vi "GameToIAStateOffensive.vi"(8 "error in (no error)":errorcluster, 11 "Game in":refnum<class "Game.lvclass">) -> (0 "error out":errorcluster, 1 "RobotRef":refnum<class "Robot.lvclass">[](array[class]), 2 "IA State out":T1={"our_robots"=[], "enemy_robots"=[], "balls"=[], "geometry"={"line_width"=0, "field_length"=0, "field_width"=0, "boundary_width"=0, "referee_width"=0, "goal_width"=0, "goal_depth"=0, "goal_wall_width"=0, "center_circle_radius"=0, "defense_radius"=0, "defense_stretch"=0, "free_kick_from_defense_dist"=0, "penalty_spot_from_field_line_dist"=0, "penalty_line_from_spot_dist"=0}, "IA Judge"={"stage"="", "command"="", "our_goalie_id"=0.0, "enemy_goalie_id"=0.0, "command enum"=enum."Halt", "Time"=enum."Azul"}, "Received Timestamp"=timestamp(0 s since 1904-01-01), "Events"={"Touch"=FALSE, "Ball out"=FALSE, "id touch"=0.0, "Ball out of \nVision"=FALSE, "Ball inside \nGoalie area"=FALSE, "Robot not responding"=FALSE, "Robots responding status"=[1.0, 1.0, 1.0, 1.0, 1.0, 1.0], "Enemy Ball \nPossession"=FALSE, "Pass State"=FALSE, "id end of pass"=0.0, "Kick"=FALSE, "Id ini Possession"=0.0, "Ball Possesion"=FALSE, "Id Possesion"=0.0, "Direct Kick"=FALSE, "2nd Strk Ativo"=FALSE}}, 3 "Game out":refnum<class "Game.lvclass">)   [LabVIEW 2018, in "Game.lvclass"]
uses:
  Game.lvclass
  Vision_class/Old vision/SSL Detection Frame Simple Estimator Cameras VelCmd Folder/Core/AI Input.ctl
  Communication_class/Paths/Convert AI Robot to Robot Command Folder/Core/AI Robot.ctl
  Communication_class/Paths/Convert AI Robot to Robot Command Folder/Intel/Functions Enum.ctl
  Communication_class/Paths/Convert AI Robot to Robot Command Folder/Intel/AttackerStates.ctl
  Communication_class/Paths/Convert AI Robot to Robot Command Folder/Path Planning/RRT/PathDests.ctl
  Communication_class/Paths/Convert AI Robot to Robot Command Folder/Path Planning/RRT/PathDest.ctl
  Communication_class/Paths/MessageAI_State Folder/Core/AI Ball.ctl
  Communication_class/Paths/MessageAI_State Folder/Core/Field Size.ctl
  Vision_class/Old vision/SSL Detection Frame Simple Estimator Cameras VelCmd Folder/Core/AI Judge.ctl
  Communication_class/Paths/MessageAI_State Folder/Intel/Command Enum.ctl
  Vision_class/Old vision/SSL Detection Frame Simple Estimator Cameras VelCmd Folder/Util/Events/Events.ctl
  Robot_class/Robot.lvclass
  Team_class/OffensivePlay.ctl
  Game.lvclass/Game.ctl
  Team_class/Team.lvclass/Team.ctl
  Object_class/Object.lvclass/Object.ctl
  Ball_class/Ball.lvclass/Ball.ctl
  Events_class/Events.lvclass/Events.ctl
  Referee_class/Referee.lvclass/Referee.ctl
  Robot_class/Robot.lvclass/Robot.ctl
  Robot_class/Read id.vi
  Object_class/Read x.vi
  Object_class/Read y.vi
  Robot_class/Read orientation.vi
  Robot_class/Read est_v_tang.vi
  Robot_class/Read est_v_norm.vi
  Object_class/Read pos_est_x.vi
  Object_class/Read pos_est_y.vi
  Robot_class/Read dribble.vi
  Robot_class/Read path.vi
  Robot_class/Read path_smooth.vi
  Robot_class/Read dest_x.vi
  Robot_class/Read dest_y.vi
  Robot_class/Read dest_orientation.vi
  Read OffensiveTeam.vi
  Read EnemyRef.vi
  Read BallRef.vi
  Read EventsRef.vi
  Read FieldRef.vi
  Read Referee.vi
  Read TimeRef.vi
  Referee_class/Read command_from_referee.vi
  Referee_class/Read command_interpreted.vi
  Events_class/Read ball_inside_enemy_goalie_area.vi
  Events_class/Read ball_inside_our_goalie_area.vi
  Events_class/Read ball_out.vi
  Events_class/Read ball_out_of_vision.vi
  Events_class/Read enemy_ball_possesion.vi
  Events_class/Read id_enemy_ball_possesion.vi
  Events_class/Read id_our_balll_possesion.vi
  Events_class/Read id_touch.vi
  Events_class/Read kick.vi
  Events_class/Read our_balll_possesion.vi
  Events_class/Read touch.vi
  Ball_class/Read v_x.vi
  Ball_class/Read v_y.vi
  Team_class/Read RobotRef.vi
  Team_class/Read OffensivePlay.vi
  Ball_class/Ball.lvclass
  Enemy_class/Enemy.lvclass
  Ally_class/Ally.lvclass
  Events_class/Events.lvclass
  Field_class/Field.lvclass
  Referee_class/Referee.lvclass
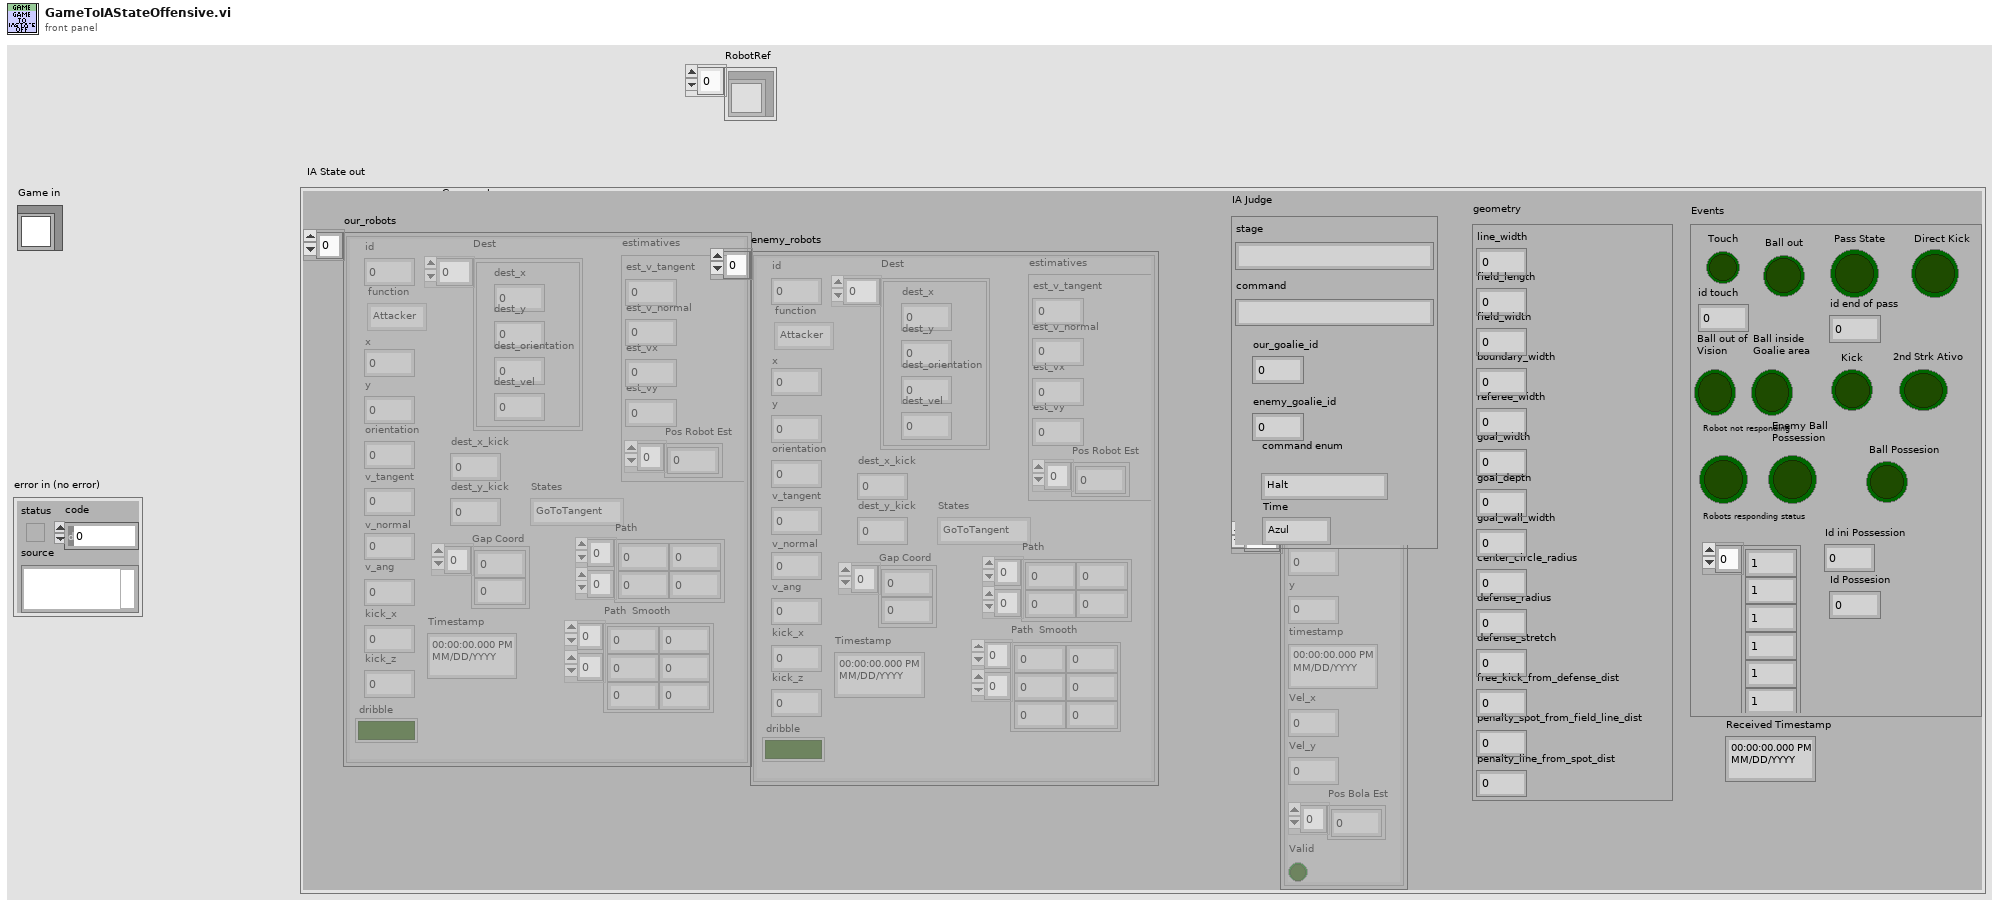
[diagram p1: front panel]
types:
  T1 = typedef "AI Input.ctl" = cluster{"our_robots":T2[], "enemy_robots":T2[], "balls":T7[], "geometry":T8, "IA Judge":T9, "Received Timestamp":timestamp, "Events":T11}
  T2 = typedef "AI Robot.ctl" = cluster{"id":u32, "function":T3, "x":dbl, "y":dbl, "orientation":dbl, "v_tangent":dbl, "v_normal":dbl, "v_ang":dbl, "kick_x":dbl, "kick_z":dbl, "dribble":bool, "Timestamp":timestamp, "estimatives":cluster{"est_v_tangent":dbl, "est_v_normal":dbl, "est_vx":dbl, "est_vy":dbl, "Pos Robot Est":dbl[]}, "dest_x_kick":dbl, "dest_y_kick":dbl, "Gap Coord":dbl[], "States":T4, "Path ":dbl[][], "Path  Smooth":dbl[][], "Dest":T5}
  T3 = typedef "Functions Enum.ctl" = enum16{"2nd Striker", "Attacker", "Goalie", "Defender", "Striker", "Goto 0", "Dummy", "Kicker", "ZigZag 0", "ZigZag 1", "ZigZag 2", "ZigZag 3", "ZigZag 4", "ZigZag 5", "ZigZag 6", "ZigZag 7", "ZigZag 8", ""}
  T4 = typedef "AttackerStates.ctl" = enum16{"Pass", "GoToTangent", "BallGetting", "GoToKick", ""}
  T5 = typedef "PathDests.ctl" = T6[]
  T6 = typedef "PathDest.ctl" = cluster{"dest_x":dbl, "dest_y":dbl, "dest_orientation":dbl, "dest_vel":dbl}
  T7 = typedef "AI Ball.ctl" = cluster{"x":dbl, "y":dbl, "timestamp":timestamp, "Vel_x":dbl, "Vel_y":dbl, "Pos Bola Est":dbl[], "Valid":bool}
  T8 = typedef "Field Size.ctl" = cluster{"line_width":u32, "field_length":u32, "field_width":u32, "boundary_width":u32, "referee_width":u32, "goal_width":u32, "goal_depth":u32, "goal_wall_width":u32, "center_circle_radius":u32, "defense_radius":u32, "defense_stretch":u32, "free_kick_from_defense_dist":u32, "penalty_spot_from_field_line_dist":u32, "penalty_line_from_spot_dist":u32}
  T9 = typedef "AI Judge.ctl" = cluster{"stage":string, "command":string, "our_goalie_id":dbl, "enemy_goalie_id":dbl, "command enum":T10, "Time":enum16{"Azul", "Amarelo"}}
  T10 = typedef "Command Enum.ctl" = enum16{"Halt", "Stop", "Force Start", "PKA Normal Start", "Prepare Kickoff Ally", "PKE Normal Start", "Prepare Kickoff Enemy", "Prepare Penalty Ally", "PPA Normal Start", "Prepare Penalty Enemy", "PPE Normal Start", "Direct Free Enemy", "Direct Free Ally", "Indirect Free Enemy", "Indirect Free Ally", "Timeout Enemy", "Timeout Ally", "Goal Enemy", "Goal Ally", "Ball Placement Enemy", "Ball Placement Ally", "Normal Half Time", "Extra Time Break", "Extra Half Time", "None", "Post Game"}
  T11 = typedef "Events.ctl" = cluster{"Touch":bool, "Ball out":bool, "id touch":dbl, "Ball out of \nVision":bool, "Ball inside \nGoalie area":bool, "Robot not responding":bool, "Robots responding status":dbl[], "Enemy Ball \nPossession":bool, "Pass State":bool, "id end of pass":dbl, "Kick":bool, "Id ini Possession":dbl, "Ball Possesion":bool, "Id Possesion":dbl, "Direct Kick":bool, "2nd Strk Ativo":bool}
  T12 = typedef "OffensivePlay.ctl" = enum16{"PreparePass", "PassToStriker", "BallOutOfField", "PassTo2ndStriker", "StopOffensive", "Prepare Penalty Enemy", "EnemyPossessionAtEnemyField", "EnemyPossesionAtOurField", "TestPlay", "PreparePenaltyAlly", "KickPenaltyAlly", "PrepareKickoffAlly", "PrepareKickoffEnemy", "IndirectEnemy", "DirectEnemy", "NormalGame", "DirectKick", "Pass", "Halt", "Timeout", "PassPlay", "PenaltyEnemy"}
  T13 = typedef "command_interpreted.ctl" = enum16{"Goal Ally", "Goal Enemy", "Ball Placement Enemy", "Ball Placement Ally", "Normal Half Time", "Extra Time  Break", "Extra Half Time", "None", "Post Game", "PKA Normal Start", "Prepare Kickoff Ally", "PKE Normal Start", "Prepare Kickoff Enemy", "Force Start", "Halt", "Timeout", "Prepare Penalty Ally", "Prepare Penalty Enemy", "PPA NormalStart", "PPE Normal Start", "Indirect Free Ally", "Direct Free Enemy", "Direct Free Ally", "Indirect Free Enemy", "Stop"}
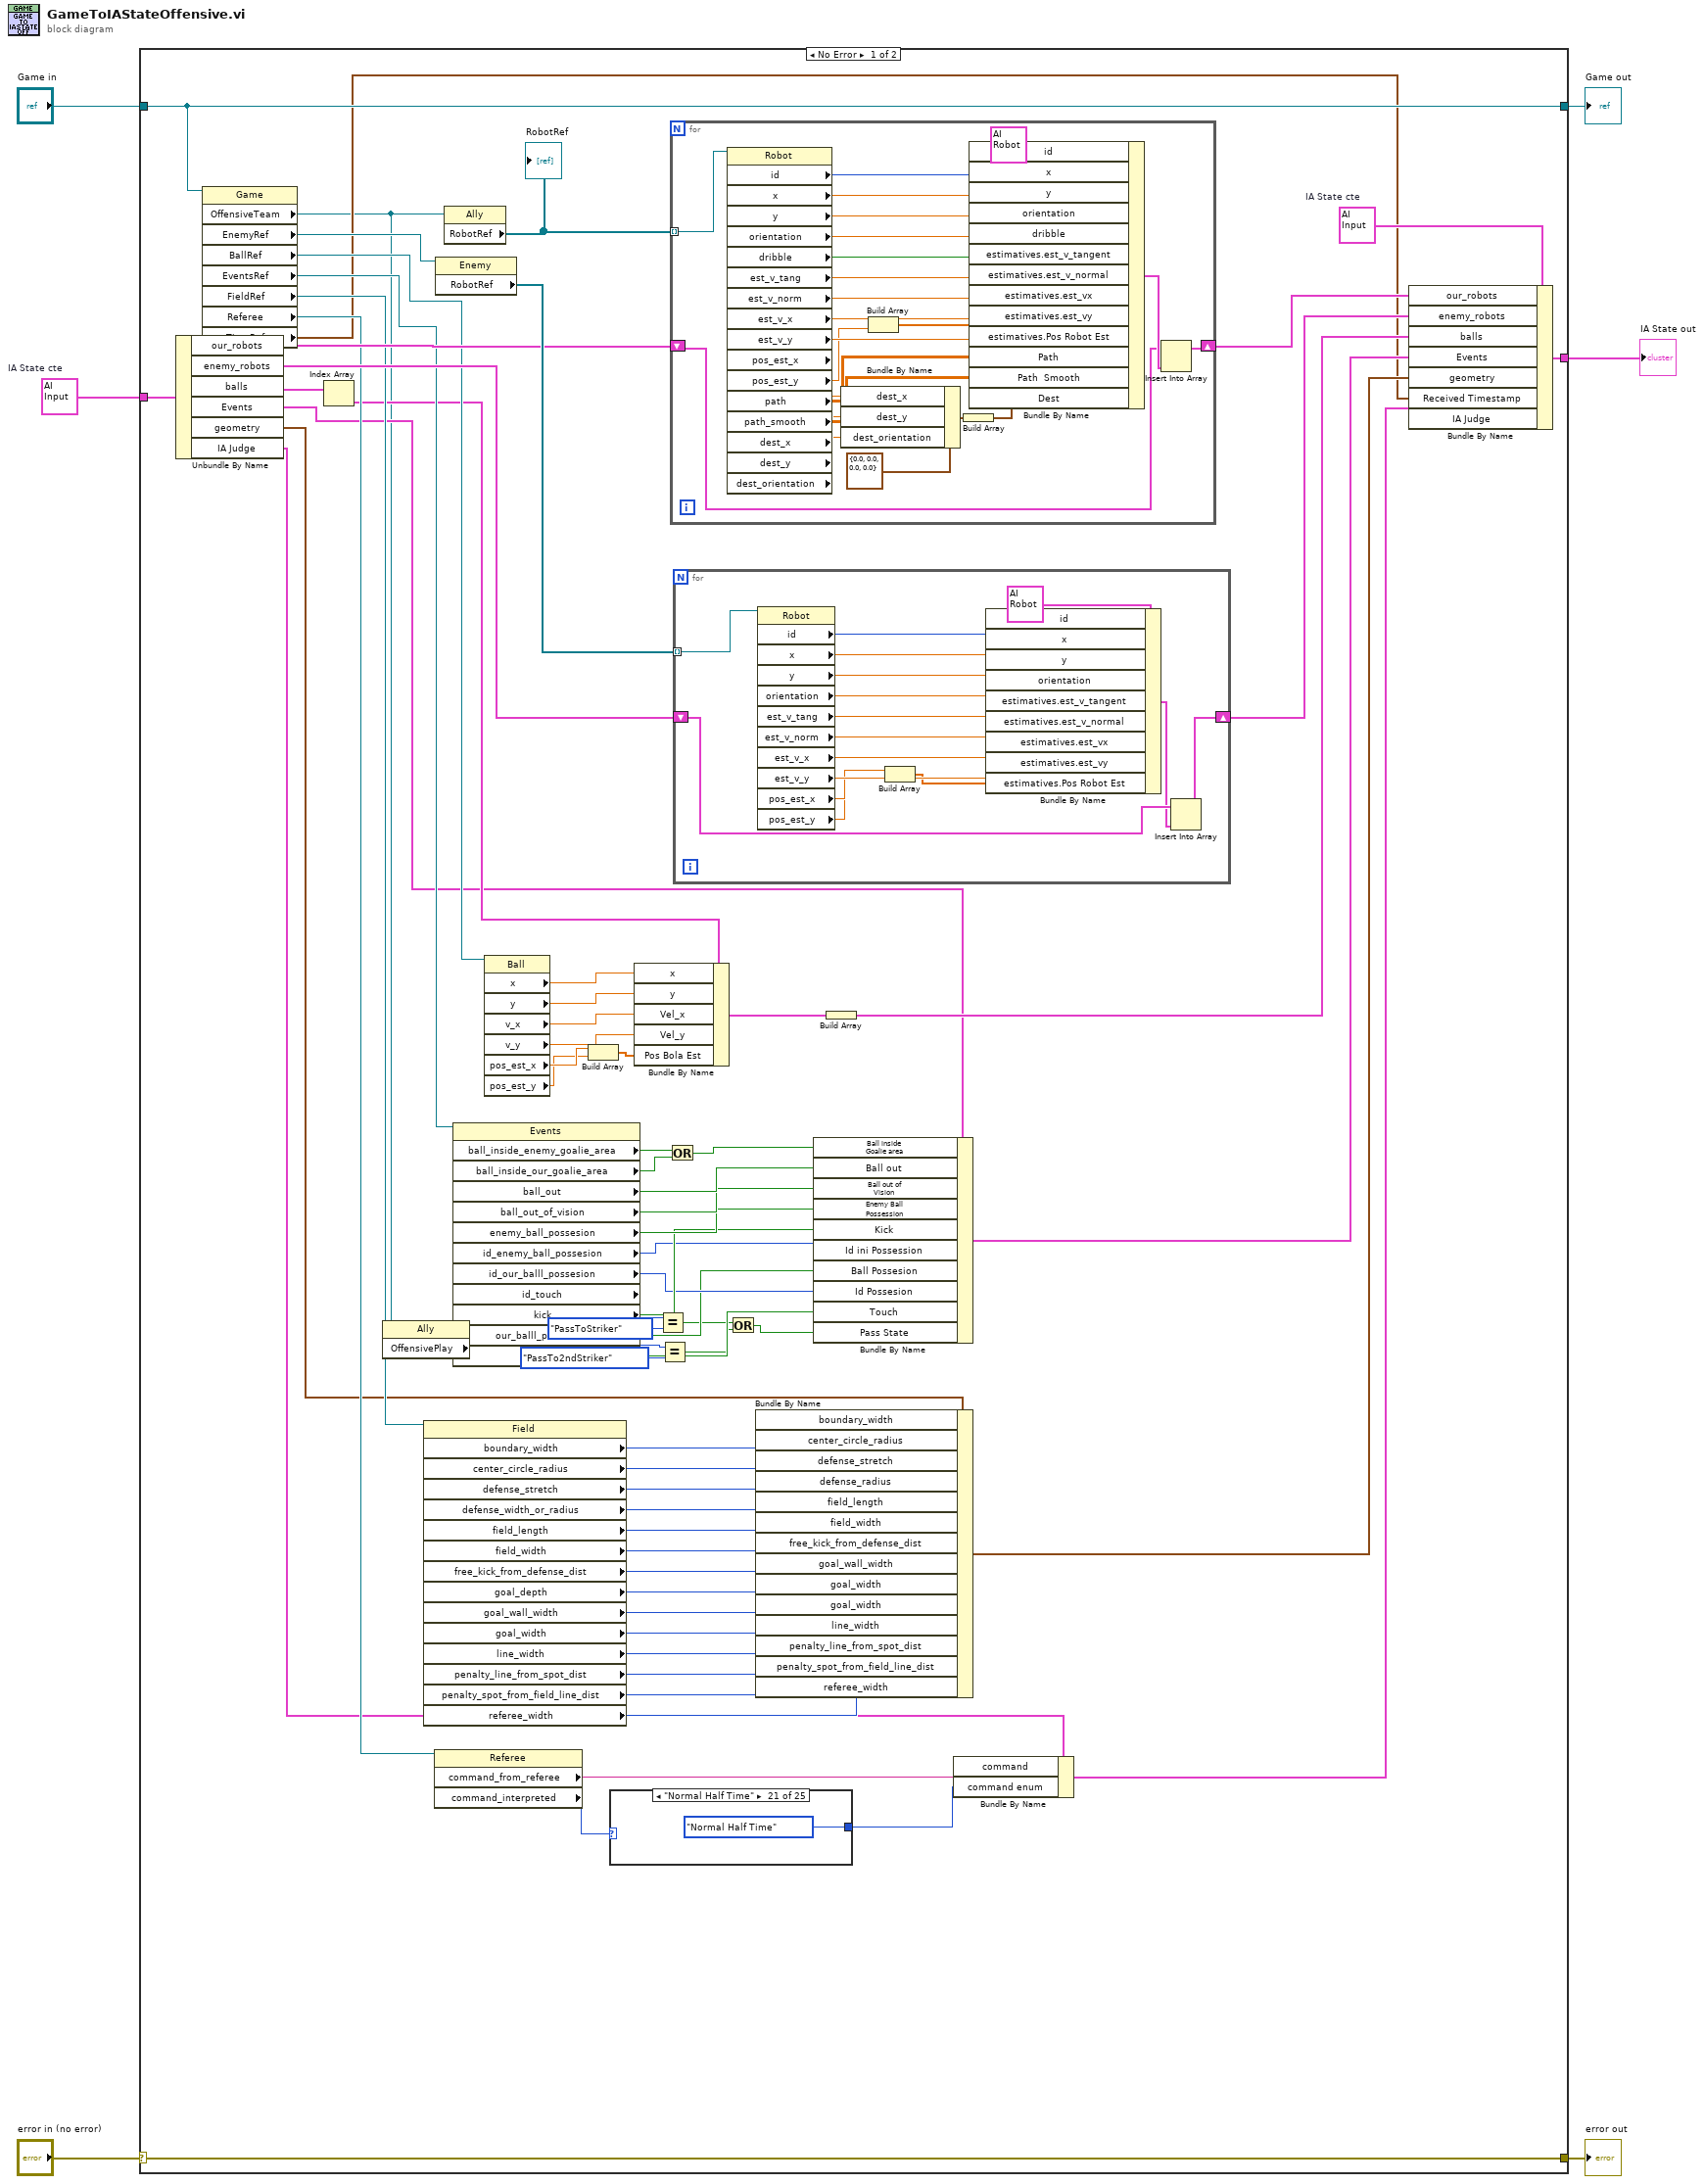
[diagram p0: block diagram]
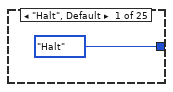
[diagram p2: hidden frame]
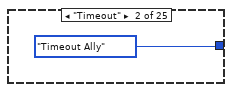
[diagram p3: hidden frame]
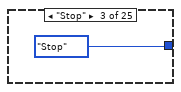
[diagram p4: hidden frame]
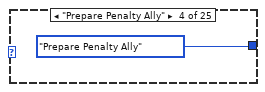
[diagram p5: hidden frame]
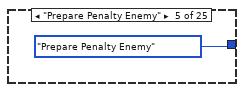
[diagram p6: hidden frame]
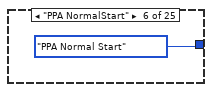
[diagram p7: hidden frame]
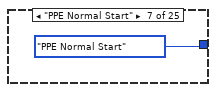
[diagram p8: hidden frame]
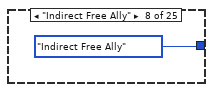
[diagram p9: hidden frame]
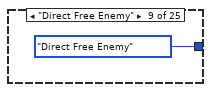
[diagram p10: hidden frame]
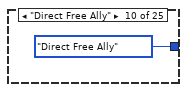
[diagram p11: hidden frame]
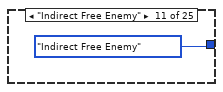
[diagram p12: hidden frame]
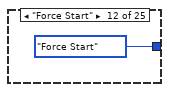
[diagram p13: hidden frame]
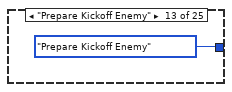
[diagram p14: hidden frame]
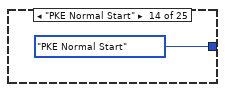
[diagram p15: hidden frame]
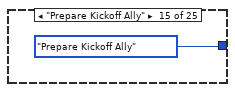
[diagram p16: hidden frame]
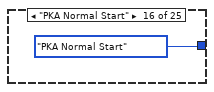
[diagram p17: hidden frame]
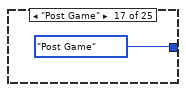
[diagram p18: hidden frame]
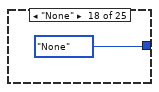
[diagram p19: hidden frame]
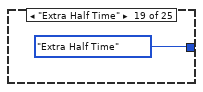
[diagram p20: hidden frame]
diagram:
  w2 = T1 {"our_robots"=[], "enemy_robots"=[], "balls"=[], "geometry"={"line_width"=0, "field_length"=0, "field_width"=0, "boundary_width"=0, "referee_width"=0, "goal_width"=0, "goal_depth"=0, "goal_wall_width"=0, "center_circle_radius"=0, "defense_radius"=0, "defense_stretch"=0, "free_kick_from_defense_dist"=0, "penalty_spot_from_field_line_dist"=0, "penalty_line_from_spot_dist"=0}, "IA Judge"={"stage"="", "command"="", "our_goalie_id"=0.0, "enemy_goalie_id"=0.0, "command enum"=enum."Halt", "Time"=enum."Azul"}, "Received Timestamp"=timestamp(0 s since 1904-01-01), "Events"={"Touch"=FALSE, "Ball out"=FALSE, "id touch"=0.0, "Ball out of \nVision"=FALSE, "Ball inside \nGoalie area"=FALSE, "Robot not responding"=FALSE, "Robots responding status"=[], "Enemy Ball \nPossession"=FALSE, "Pass State"=FALSE, "id end of pass"=0.0, "Kick"=FALSE, "Id ini Possession"=0.0, "Ball Possesion"=FALSE, "Id Possesion"=0.0, "Direct Kick"=FALSE, "2nd Strk Ativo"=FALSE}}  # IA State cte
  n1 = case shown="No Error" "error in (no error)" {
    selector: "error in (no error)" -> [w75 w144]
    tunnel: [w75 w144] -> w5
    tunnel: [w74 w143] -> w3
    tunnel: "Game in" -> [w74 w143]
    tunnel: w2 -> [w70 w142]
    tunnel: [w14 w142] -> w1
    frame No Error {
      w66 = T1 {"our_robots"=[], "enemy_robots"=[], "balls"=[], "geometry"={"line_width"=0, "field_length"=0, "field_width"=0, "boundary_width"=0, "referee_width"=0, "goal_width"=0, "goal_depth"=0, "goal_wall_width"=0, "center_circle_radius"=0, "defense_radius"=0, "defense_stretch"=0, "free_kick_from_defense_dist"=0, "penalty_spot_from_field_line_dist"=0, "penalty_line_from_spot_dist"=0}, "IA Judge"={"stage"="", "command"="", "our_goalie_id"=0.0, "enemy_goalie_id"=0.0, "command enum"=enum."Halt", "Time"=enum."Azul"}, "Received Timestamp"=timestamp(0 s since 1904-01-01), "Events"={"Touch"=FALSE, "Ball out"=FALSE, "id touch"=0.0, "Ball out of \nVision"=FALSE, "Ball inside \nGoalie area"=FALSE, "Robot not responding"=FALSE, "Robots responding status"=[], "Enemy Ball \nPossession"=FALSE, "Pass State"=FALSE, "id end of pass"=0.0, "Kick"=FALSE, "Id ini Possession"=0.0, "Ball Possesion"=FALSE, "Id Possesion"=0.0, "Direct Kick"=FALSE, "2nd Strk Ativo"=FALSE}}  # IA State cte
      n2 = Unbundle By Name(w70) -> ("our_robots"=w69:T2[], "enemy_robots"=w68:T2[], "balls"=w23:T7[], "Events"=w21:T11, "geometry"=w20:T8, "IA Judge"=w18:T9)
      n3 = property class="Game"(reference=w74) -> ("OffensiveTeam"=w13:refnum<class "Ally.lvclass">, "EnemyRef"=w72:refnum<class "Enemy.lvclass">, "BallRef"=w67:refnum<class "Ball.lvclass">, "EventsRef"=w54:refnum<class "Events.lvclass">, "FieldRef"=w41:refnum<class "Field.lvclass">, "Referee"=w25:refnum<class "Referee.lvclass">, "TimeRef"=w19:timestamp)  [unwired: 1 in, 2 out]
      n4 = Index Array(array=w23) -> (element=w22:T7)  [unwired: 1 in]
      n5 = property class="Ally"(reference=w13) -> ("OffensivePlay"=w9:T12)  [unwired: 1 in, 2 out]
      n6 = property class="Field"(reference=w41) -> ("boundary_width"=w40:i32, "center_circle_radius"=w39:i32, "defense_stretch"=w38:i32, "defense_width_or_radius"=w37:i32, "field_length"=w36:i32, "field_width"=w35:i32, "free_kick_from_defense_dist"=w34:i32, "goal_depth"=w33:i32, "goal_wall_width"=w32:i32, "goal_width"=w31:i32, "line_width"=w30:i32, "penalty_line_from_spot_dist"=w29:i32, "penalty_spot_from_field_line_dist"=w28:i32, "referee_width"=w27:i32)  [unwired: 1 in, 2 out]
      n7 = property class="Referee"(reference=w25) -> ("command_from_referee"=w24:string, "command_interpreted"=w17:T13)  [unwired: 1 in, 2 out]
      n8 = property class="Enemy"(reference=w72) -> ("RobotRef"=w71:refnum<class "Robot.lvclass">[])  [unwired: 1 in, 2 out]
      n9 = property class="Ally"(reference=w13) -> ("RobotRef"=w73:refnum<class "Robot.lvclass">[])  [unwired: 1 in, 2 out]
      "RobotRef" <- w73
      n10 = property class="Events" props=["ball_inside_enemy_goalie_area", "ball_inside_our_goalie_area", "ball_out", "ball_out_of_vision", "enemy_ball_possesion", "id_enemy_ball_possesion", "id_our_balll_possesion", "id_touch", "kick", "our_balll_possesion", "touch"](reference=w54) -> ("ball_inside_enemy_goalie_area"=w52:bool, "ball_inside_our_goalie_area"=w53:bool, "ball_out"=w50:bool, "ball_out_of_vision"=w49:bool, "enemy_ball_possesion"=w48:bool, "id_enemy_ball_possesion"=w46:i32, "id_our_balll_possesion"=w45:i32, "kick"=w47:bool, "our_balll_possesion"=w44:bool, "touch"=w43:bool)  [unwired: 1 in, 3 out]
      n11 = property class="Ball"(reference=w67) -> ("x"=w63:dbl, "y"=w62:dbl, "v_x"=w61:dbl, "v_y"=w60:dbl, "pos_est_x"=w59:dbl, "pos_est_y"=w58:dbl)  [unwired: 1 in, 2 out]
      n12 = Build Array(w59, w58) -> (w57:dbl[])
      n13 = case shown="\"Normal Half Time\"" w17 {
        tunnel: [Command_Enum."Halt" ("command enum") Command_Enum."Timeout Ally" ("command enum") Command_Enum."Stop" ("command enum") Command_Enum."Prepare Penalty Ally" ("command enum") Command_Enum."Prepare Penalty Enemy" ("command enum") Command_Enum."PPA Normal Start" ("command enum") Command_Enum."PPE Normal Start" ("command enum") Command_Enum."Indirect Free Ally" ("command enum") Command_Enum."Direct Free Enemy" ("command enum") Command_Enum."Direct Free Ally" ("command enum") Command_Enum."Indirect Free Enemy" ("command enum") Command_Enum."Force Start" ("command enum") Command_Enum."Prepare Kickoff Enemy" ("command enum") Command_Enum."PKE Normal Start" ("command enum") Command_Enum."Prepare Kickoff Ally" ("command enum") Command_Enum."PKA Normal Start" ("command enum") Command_Enum."Post Game" ("command enum") Command_Enum."None" ("command enum") Command_Enum."Extra Half Time" ("command enum") Command_Enum."Extra Time Break" ("command enum") Command_Enum."Normal Half Time" ("command enum") Command_Enum."Ball Placement Ally" ("command enum") Command_Enum."Ball Placement Enemy" ("command enum") Command_Enum."Goal Enemy" ("command enum") Command_Enum."Goal Ally" ("command enum")] -> w16
        frame "Halt", Default {
        }
        frame "Timeout" {
        }
        frame "Stop" {
        }
        frame "Prepare Penalty Ally" {
        }
        frame "Prepare Penalty Enemy" {
        }
        frame "PPA NormalStart" {
        }
        frame "PPE Normal Start" {
        }
        frame "Indirect Free Ally" {
        }
        frame "Direct Free Enemy" {
        }
        frame "Direct Free Ally" {
        }
        frame "Indirect Free Enemy" {
        }
        frame "Force Start" {
        }
        frame "Prepare Kickoff Enemy" {
        }
        frame "PKE Normal Start" {
        }
        frame "Prepare Kickoff Ally" {
        }
        frame "PKA Normal Start" {
        }
        frame "Post Game" {
        }
        frame "None" {
        }
        frame "Extra Half Time" {
        }
        frame "Extra Time  Break" {
        }
        frame "Normal Half Time" {
        }
        frame "Ball Placement Ally" {
        }
        frame "Ball Placement Enemy" {
        }
        frame "Goal Enemy" {
        }
        frame "Goal Ally" {
        }
      }
      n14 = Bundle By Name(cluster=w22, "x"=w63, "y"=w62, "Vel_x"=w61, "Vel_y"=w60, "Pos Bola Est"=w57) -> (w56:T7)
      n15 = Equal?(x=w9, y=OffensivePlay."PassToStriker") -> (x = y?=w11:bool)
      n16 = Equal?(x=w9, y=OffensivePlay."PassTo2ndStriker") -> (x = y?=w8:bool)
      n17 = Or(x=w52, y=w53) -> (x .or. y?=w51:bool)
      n18 = for {
        tunnel: w73 -> [w121] mode=indexing
        shift-right: [w122] -> w65
        shift-left: w69 -> [w123]
        n19 = property class="Robot"(reference=w121) -> ("id"=w120:i32, "x"=w119:dbl, "y"=w118:dbl, "orientation"=w117:dbl, "dribble"=w116:bool, "est_v_tang"=w115:dbl, "est_v_norm"=w114:dbl, "est_v_x"=w113:dbl, "est_v_y"=w112:dbl, "pos_est_x"=w111:dbl, "pos_est_y"=w110:dbl, "path"=w108:dbl[][], "path_smooth"=w107:dbl[][], "dest_x"=w106:dbl, "dest_y"=w105:dbl, "dest_orientation"=w104:dbl)  [unwired: 1 in, 2 out]
        n20 = Bundle By Name(cluster=T6 {"dest_x"=0.0, "dest_y"=0.0, "dest_orientation"=0.0, "dest_vel"=0.0} ("element"), "dest_x"=w106, "dest_y"=w105, "dest_orientation"=w104) -> (w102:T6)
        n21 = Build Array(w111, w110) -> (w109:dbl[])
        n22 = Build Array(w102) -> (w101:T6[])
        n23 = Bundle By Name(cluster=T2 {"id"=0, "function"=enum."Attacker", "x"=0.0, "y"=0.0, "orientation"=0.0, "v_tangent"=0.0, "v_normal"=0.0, "v_ang"=0.0, "kick_x"=0.0, "kick_z"=0.0, "dribble"=FALSE, "Timestamp"=timestamp(0 s since 1904-01-01), "estimatives"={"est_v_tangent"=0.0, "est_v_normal"=0.0, "est_vx"=0.0, "est_vy"=0.0, "Pos Robot Est"=[]}, "dest_x_kick"=0.0, "dest_y_kick"=0.0, "Gap Coord"=[], "States"=enum."GoToTangent", "Path "=[], "Path  Smooth"=[], "Dest"=[]} ("Robot"), "id"=w120, "x"=w119, "y"=w118, "orientation"=w117, "dribble"=w116, "estimatives.est_v_tangent"=w115, "estimatives.est_v_normal"=w114, "estimatives.est_vx"=w113, "estimatives.est_vy"=w112, "estimatives.Pos Robot Est"=w109, "Path"=w108, "Path  Smooth"=w107, "Dest"=w101) -> (w124:T2)
        n24 = Insert Into Array(array=w123, new element=w124) -> (w122:T2[])  [unwired: 1 in]
      }
      n25 = for {
        tunnel: w71 -> [w136] mode=indexing
        shift-right: [w126] -> w64
        shift-left: w68 -> [w135]
        n26 = property class="Robot"(reference=w136) -> ("id"=w138:i32, "x"=w139:dbl, "y"=w140:dbl, "orientation"=w141:dbl, "est_v_tang"=w134:dbl, "est_v_norm"=w133:dbl, "est_v_x"=w132:dbl, "est_v_y"=w131:dbl, "pos_est_x"=w130:dbl, "pos_est_y"=w129:dbl)  [unwired: 1 in, 2 out]
        n27 = Build Array(w130, w129) -> (w128:dbl[])
        n28 = Bundle By Name(cluster=T2 {"id"=0, "function"=enum."Attacker", "x"=0.0, "y"=0.0, "orientation"=0.0, "v_tangent"=0.0, "v_normal"=0.0, "v_ang"=0.0, "kick_x"=0.0, "kick_z"=0.0, "dribble"=FALSE, "Timestamp"=timestamp(0 s since 1904-01-01), "estimatives"={"est_v_tangent"=0.0, "est_v_normal"=0.0, "est_vx"=0.0, "est_vy"=0.0, "Pos Robot Est"=[]}, "dest_x_kick"=0.0, "dest_y_kick"=0.0, "Gap Coord"=[], "States"=enum."GoToTangent", "Path "=[], "Path  Smooth"=[], "Dest"=[]} ("Robot"), "id"=w138, "x"=w139, "y"=w140, "orientation"=w141, "estimatives.est_v_tangent"=w134, "estimatives.est_v_normal"=w133, "estimatives.est_vx"=w132, "estimatives.est_vy"=w131, "estimatives.Pos Robot Est"=w128) -> (w127:T2)
        n29 = Insert Into Array(array=w135, new element=w127) -> (w126:T2[])  [unwired: 1 in]
      }
      n30 = Or(x=w11, y=w8) -> (x .or. y?=w7:bool)
      n31 = Bundle By Name(cluster=w20, "boundary_width"=w40, "center_circle_radius"=w39, "defense_stretch"=w38, "defense_radius"=w37, "field_length"=w36, "field_width"=w35, "free_kick_from_defense_dist"=w34, "goal_wall_width"=w33, "goal_width"=w32, "goal_width"=w31, "line_width"=w30, "penalty_line_from_spot_dist"=w29, "penalty_spot_from_field_line_dist"=w28, "referee_width"=w27) -> (w26:T8)
      n32 = Bundle By Name(cluster=w21, "Ball inside \nGoalie area"=w51, "Ball out"=w50, "Ball out of \nVision"=w49, "Enemy Ball \nPossession"=w48, "Kick"=w47, "Id ini Possession"=w46, "Ball Possesion"=w44, "Id Possesion"=w45, "Touch"=w43, "Pass State"=w7) -> (w42:T11)
      n33 = Build Array(w56) -> (w55:T7[])
      n34 = Bundle By Name(cluster=w18, "command"=w24, "command enum"=w16) -> (w15:T9)
      n35 = Bundle By Name(cluster=w66, "our_robots"=w65, "enemy_robots"=w64, "balls"=w55, "Events"=w42, "geometry"=w26, "Received Timestamp"=w19, "IA Judge"=w15) -> (w14:T1)
    }
    frame Error {
    }
  }
  "error out" <- w5
  "Game out" <- w3
  "IA State out" <- w1
